vi "Calcu_Air density.vi"() -> (2 "t(℃)":dbl, 3 "ρ_air":dbl)   [LabVIEW 2020]
uses:
  Variables/Global_Cal Info.vi
  <vilib>/express/express arith-compare/Formula/XNode/ExpressFormulaBlockNode.xnode
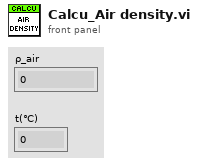
[diagram p1: front panel]
types:
  T1 = typedef "Clst_Atm Info Global.ctl" = cluster{"교정장소":enum16{"0 : 고정표준실", "1 : 현장교정"}, "최저온도(℃)":string, "최고온도(℃)":string, "최저습도(％ R.H.)":string, "최고습도(％ R.H.)":string, "최저기압(hPa)":string, "최고기압(hPa)":string, "교정실명":string}
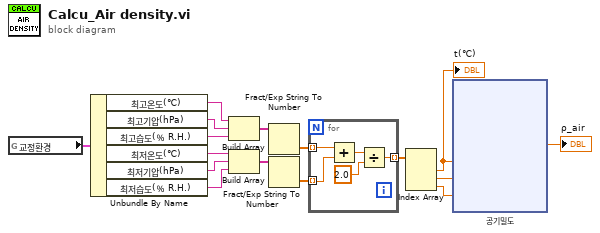
[diagram p0: block diagram]
diagram:
  n1 = global read "Global_Cal Info.vi" "교정환경"() -> (w14:T1)
  n2 = Unbundle By Name(w14) -> ("최고온도(℃)"=w6:string, "최고기압(hPa)"=w5:string, "최고습도(％ R.H.)"=w3:string, "최저온도(℃)"=w4:string, "최저기압(hPa)"=w13:string, "최저습도(％ R.H.)"=w12:string)
  n3 = Build Array(w6, w5, w3) -> (w2:string[])
  n4 = Build Array(w4, w13, w12) -> (w1:string[])
  n5 = Fract/Exp String To Number(string=w2) -> (number=w11:dbl[])  [unwired: 3 in, 1 out]
  n6 = Fract/Exp String To Number(string=w1) -> (number=w10:dbl[])  [unwired: 3 in, 1 out]
  n7 = for {
    tunnel: w11 -> [w21] mode=indexing
    tunnel: w10 -> [w20] mode=indexing
    tunnel: [w17] -> w9 mode=indexing
    n8 = Add(x=w21, y=w20) -> (x+y=w19:dbl)
    n9 = Divide(x=w19, y=2.0) -> (x/y=w17:dbl)
  }
  n10 = Index Array(array=w9) -> (element #1=w16:dbl, element #2=w8:dbl, element #3=w7:dbl)  [unwired: 3 in]
  "t(℃)" <- w16
  n11 = xnode ("공기밀도")("t"=w16, "p"=w8, "h"=w7) -> ("결과"=→"ρ_air":dbl)  [unwired: 1 in, 1 out]
